vi "Read Key (Boolean).vi"(7 "section":string, 8 "error in (no error)":errorcluster, 9 "default value":bool, 10 "key":string, 11 "refnum":T1) -> (0 "error out":errorcluster, 1 "value":bool, 2 "found?":bool, 3 "refnum out":T1)   [LabVIEW 2010, in "NI_LVConfig.lvlib"]
doc: "Reads a value associated with a key in a specified section from the configuration data identified by <B>refnum</B>. If the key does not exist, the VI returns the default value. This VI supports multibyte characters in strings. Wire data to the <B>default value</B> input to determine the polymorphic instance to use or manually select the instance."
uses:
  NI_LVConfig.lvlib
  Config Data RefNum.ctl
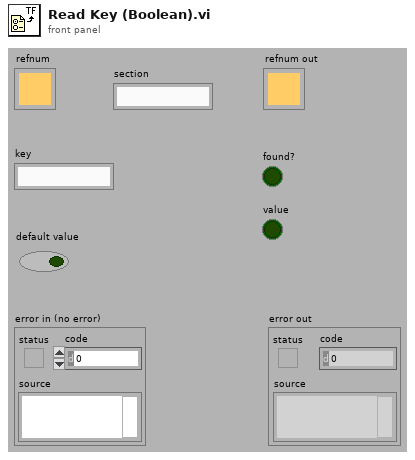
[diagram p1: front panel]
types:
  T1 = typedef "NI_LVConfig.lvlib/Config Data RefNum.ctl" = refnum<k1>
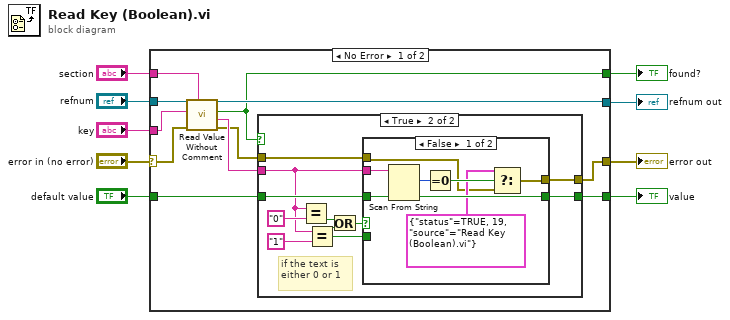
[diagram p0: block diagram]
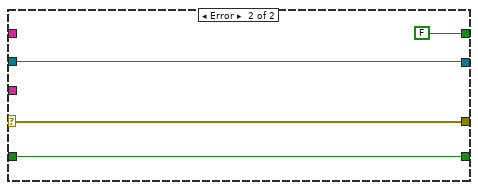
[diagram p4: hidden frame]
diagram:
  n1 = case shown="No Error" "error in (no error)" {
    selector: "error in (no error)" -> [w13 w46]
    tunnel: [w19 w46] -> w8
    tunnel: [w17 w43] -> w2
    tunnel: "section" -> [w12 _]
    tunnel: "key" -> [w11 _]
    tunnel: "default value" -> [w18 w45]
    tunnel: [w20 w45] -> w4
    tunnel: [w16 FALSE ("key exists?")] -> w3
    tunnel: "refnum" -> [w10 w43]
    frame No Error {
      n2 = call "Read Value Without Comment.vi"("section"=w12, "error in (no error)"=w13, "key"=w11, "refnum"=w10) -> ("error out"=w14:errorcluster, "value"=w15:string, "found?"=w16:bool, "refnum out"=w17:T1)  [unwired: 4 out]
      n3 = case shown="True" w16 {
        tunnel: [w22 w32] -> w20
        tunnel: w18 -> [w22 w31]
        tunnel: w15 -> [_ w23]
        tunnel: w14 -> [w21 w25]
        tunnel: [w21 w24] -> w19
        frame False {
        }
        frame True {
          # "if the text is either 0 or 1"
          n4 = Equal?(x=w23, y="0") -> (x = y?=w27:bool)
          n5 = Equal?(x=w23, y="1") -> (x = y?=w28:bool)
          n6 = Or(x=w27, y=w28) -> (x .or. y?=w26:bool)
          n7 = case shown="False" w26 {
            tunnel: [w40 w42] -> w32
            tunnel: w23 -> [w39 _]
            tunnel: w31 -> [w38 _]
            tunnel: w28 -> [_ w42]
            tunnel: w25 -> [w33 w41]
            tunnel: [w35 w41] -> w24
            frame False {
              n8 = Scan From String(input string=w39, default 1=w38) -> (offset past scan=w37:u32, output 1=w40:bool)  [unwired: 3 in, 2 out]
              n9 = Equal To 0?(x=w37) -> (x = 0?=w36:bool)
              n10 = Select(t=cluster{"status":bool, u16, "source":string} {"status"=TRUE, 19, "source"="Read Key (Boolean).vi"} ("f"), s=w36, f=w33) -> (s? t:f=w35:errorcluster)
            }
            frame True {
            }
          }
        }
      }
    }
    frame Error {
    }
  }
  "error out" <- w8
  "found?" <- w3
  "value" <- w4
  "refnum out" <- w2
